vi "PolyFitQuery.vi"(0 "Utilities in":refnum<class "Utilities.lvclass">, 1 "Coefficients":dbl[](array[numeric]), 5 "x":dbl, 7 "y":dbl, 9 "z":dbl, 11 "error in (no error)":errorcluster) -> (4 "Utilities out":refnum<class "Utilities.lvclass">, 8 "f(x, y, z)":dbl format="%.2f", 15 "error out":errorcluster)   [LabVIEW 2023, in "Utilities.lvclass"]
uses:
  Utilities.lvclass
  <vilib>/Analysis/baseanly.llb/Real Dot Product.vi
  <vilib>/Analysis/NI_AALBase.lvlib
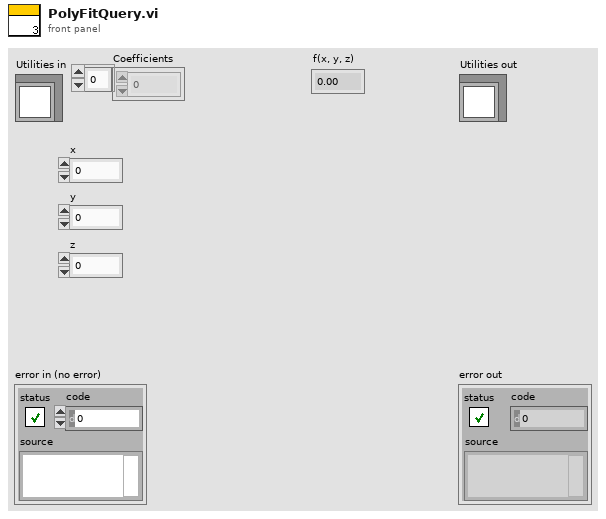
[diagram p1: front panel]
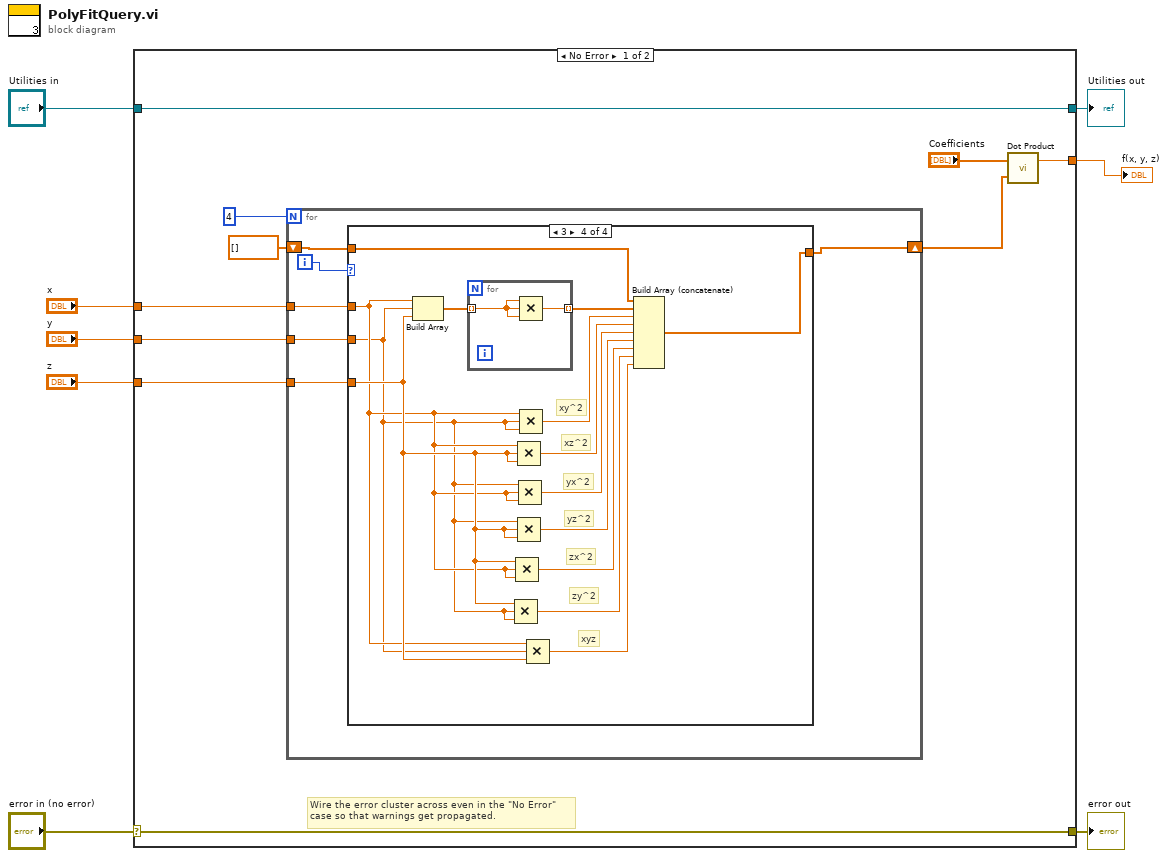
[diagram p0: block diagram]
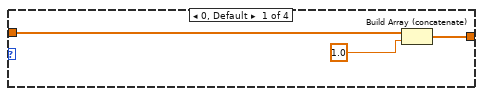
[diagram p2: hidden frame]
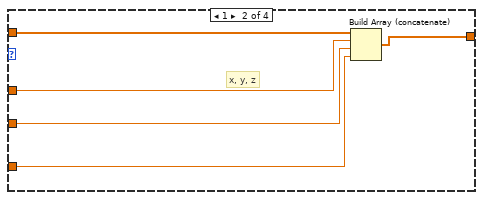
[diagram p3: hidden frame]
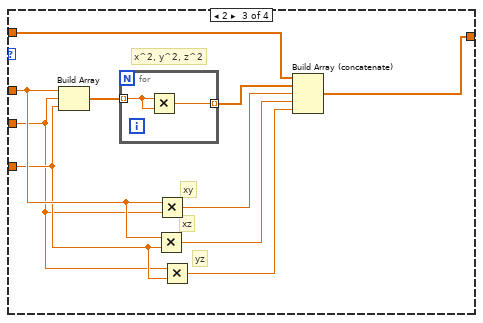
[diagram p4: hidden frame]
diagram:
  n1 = case shown="No Error" "error in (no error)" {
    selector: "error in (no error)" -> [w17 w62]
    tunnel: [w17 w62] -> w7
    tunnel: [w18 w61] -> w5
    tunnel: "Utilities in" -> [w18 w61]
    tunnel: "x" -> [w15 _]
    tunnel: "y" -> [w14 _]
    tunnel: "z" -> [w13 _]
    tunnel: [w9 _] -> w1
    frame No Error {
      # "Wire the error cluster across even in the \"No Error\"\ncase so that warnings get propagated."
      n2 = for {
        N: 4 -> [_]
        tunnel: w15 -> [w23]
        tunnel: w14 -> [w22]
        shift-right: [w19] -> w10
        shift-left: dbl[] [] -> [w20]
        tunnel: w13 -> [w21]
        i -> [w24]
        n3 = case shown="3" w24 {
          tunnel: w23 -> [_ w31 w39 w47]
          tunnel: w22 -> [_ w30 w37 w46]
          tunnel: w21 -> [_ w29 w38 w48]
          tunnel: w20 -> [w27 w32 w41 w45]
          tunnel: [w26 w28 w33 w58] -> w19
          frame 0, Default {
            n4 = Build Array (concatenate)(w27, 1.0 ("element")) -> (w26:dbl[])
          }
          frame 1 {
            # "x, y, z"
            n5 = Build Array (concatenate)(w32, w31, w30, w29) -> (w28:dbl[])
          }
          frame 2 {
            # "yz"
            # "xz"
            # "xy"
            # "x^2, y^2, z^2"
            n6 = Build Array(w39, w37, w38) -> (w42:dbl[])
            n7 = for {
              tunnel: w42 -> [w44] mode=indexing
              tunnel: [w43] -> w40 mode=indexing
              n8 = Multiply(x=w44, y=w44) -> (x*y=w43:dbl)
            }
            n9 = Multiply(x=w39, y=w38) -> (x*y=w35:dbl)
            n10 = Multiply(x=w39, y=w37) -> (x*y=w36:dbl)
            n11 = Multiply(x=w37, y=w38) -> (x*y=w34:dbl)
            n12 = Build Array (concatenate)(w41, w40, w36, w35, w34) -> (w33:dbl[])
          }
          frame 3 {
            # "xyz"
            # "zy^2"
            # "zx^2"
            # "yz^2"
            # "yx^2"
            # "xz^2"
            # "xy^2"
            n13 = Build Array(w47, w46, w48) -> (w57:dbl[])
            n14 = for {
              tunnel: w57 -> [w60] mode=indexing
              tunnel: [w59] -> w51 mode=indexing
              n15 = Compound Arithmetic op=MULTIPLY(w60, w60, w60) -> (w59:dbl)
            }
            n16 = Compound Arithmetic op=MULTIPLY(w48, w46, w46) -> (w55:dbl)
            n17 = Compound Arithmetic op=MULTIPLY(w48, w47, w47) -> (w54:dbl)
            n18 = Compound Arithmetic op=MULTIPLY(w47, w48, w48) -> (w50:dbl)
            n19 = Compound Arithmetic op=MULTIPLY(w46, w48, w48) -> (w53:dbl)
            n20 = Compound Arithmetic op=MULTIPLY(w46, w47, w47) -> (w52:dbl)
            n21 = Compound Arithmetic op=MULTIPLY(w47, w46, w46) -> (w49:dbl)
            n22 = Compound Arithmetic op=MULTIPLY(w47, w46, w48) -> (w56:dbl)
            n23 = Build Array (concatenate)(w45, w51, w49, w50, w52, w53, w54, w55, w56) -> (w58:dbl[])
          }
        }
      }
      n24 = call-poly <vilib>:"Dot Product.vi"("Y Vector"=w10, "X Vector"="Coefficients") -> ("X * Y"=w9:dbl)  [unwired: 1 out]
    }
    frame Error {
    }
  }
  "error out" <- w7
  "Utilities out" <- w5
  "f(x, y, z)" <- w1
